vi "Enable All Loggers.vi"(8 "error in":errorcluster) -> (0 "error out":errorcluster)   [LabVIEW 2018, in "Logging.lvlib"]
uses:
  Logging.lvlib
  Registry/Registry.lvlib
panel:
  # "Connector Pane"
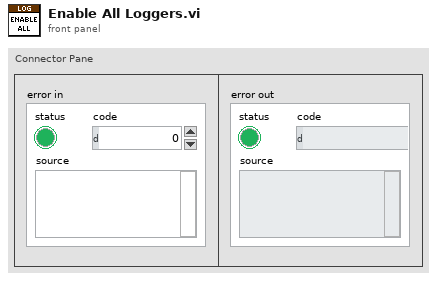
[diagram p1: front panel]
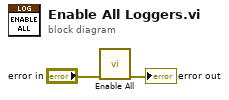
[diagram p0: block diagram]
diagram:
  n1 = call "Enable All.vi"("error in"="error in") -> ("error out"=→"error out":errorcluster)  [unwired: 10 in]
